vi "Facade.vi"(0 "Data In":T7 {"Duration (s)" format="%<%M:%S>T"}, 2 "Display State In":T5, 3 "Container State":T6) -> (6 "Data Out":T7 {"Duration (s)" format="%<%M:%S>T"}, 7 "Display State Out":T5, 8 "Action":T4)   [LabVIEW 2015, in "Artist Browser.lvlib" / "Artist Browser.xctl"]
uses:
  Artist Browser.xctl
  Data.ctl
  controls/Music Library Element Display.ctl
  file/MusicElement/Song/Song Duration.ctl
  <vilib>/_xctls/Container State.ctl
  State.ctl
  <vilib>/_xctls/Action.ctl
  controls/Ascending_Descending Order.ctl
  file/MusicElement/MusicElementLibrary/MusicLibrary/Music Library Sort Option.ctl
  <vilib>/_xctls/XControlSupport.lvlib
  file/MusicElement/MusicElementLibrary/MusicLibrary/MusicLibrary.lvclass
  file/MusicElement/Song/Song.lvclass
panel:
  out "Unfiltered Array":T1[](array[typedef]) {"Duration (s)" format="%<%M:%S>T"}
  in  "Remove Filters":bool
  in  "Time Sort":bool
  out "Sort Time Indicator":T3
  out "Sort Artist Indicator":T3
  in  "Artist Sort":bool
  in  "Song Sort":bool
  out "Sort Songs Indicator":T3
  in  "Array":T1[](array[typedef]) {"Duration (s)" format="%<%M:%S>T"}
  in  "Scrollbar":i32(c297)
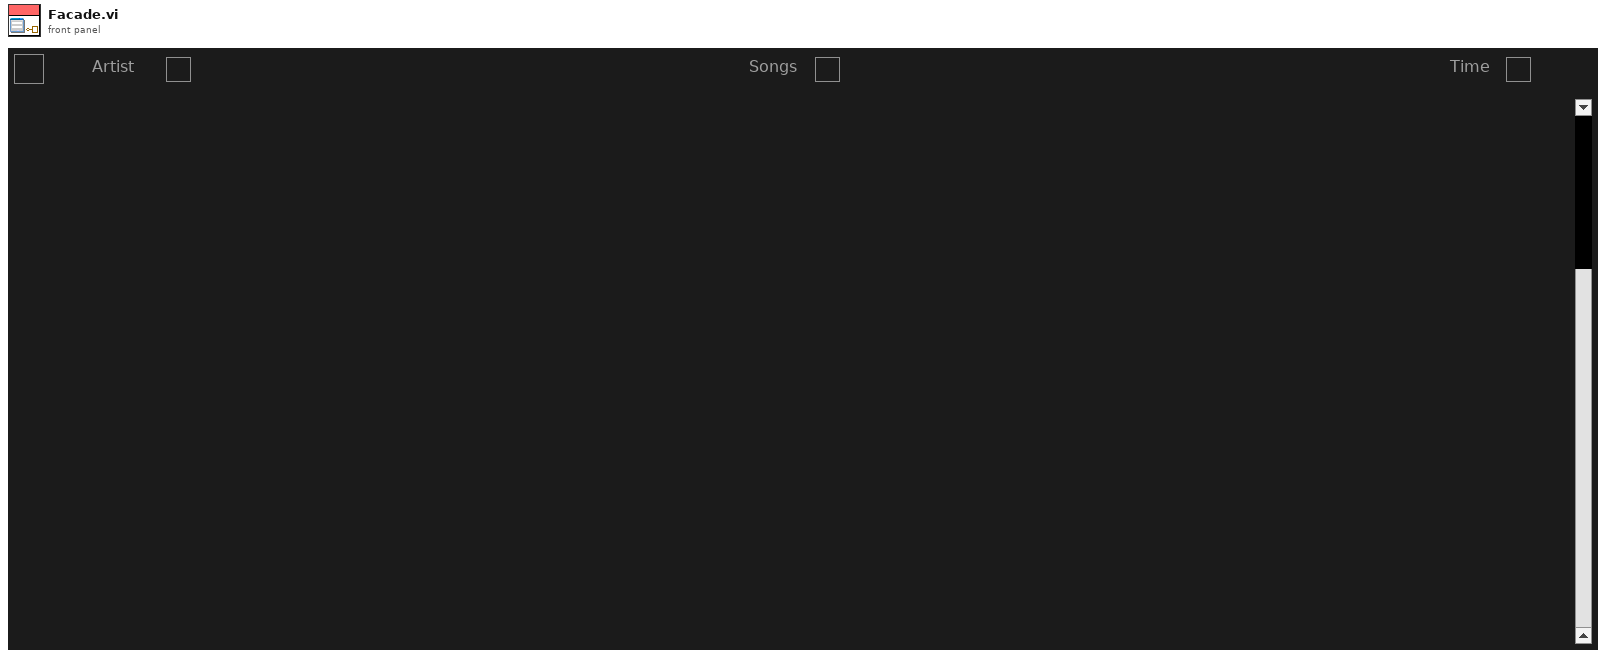
[diagram p1: front panel]
types:
  T1 = typedef "Music Library Element Display.ctl" = cluster{"Name":string, "Details":string, "Duration (s)":T2, "Click":bool}
  T2 = typedef "Song.lvclass/Song Duration.ctl" = timestamp
  T3 = typedef "Ascending_Descending Order.ctl" = bool
  T4 = typedef "XControlSupport.lvlib/Action.ctl" = cluster{"Data Changed?":bool, "State Changed?":bool, "Action Name":string}
  T5 = typedef "Artist Browser.lvlib/Artist Browser.xctl/State.ctl" = cluster{"Event - Element Selected":refnum<user-event>}
  T6 = typedef "XControlSupport.lvlib/Container State.ctl" = cluster{"Indicator?":bool, "Run Mode?":bool, " Refnum":refnum<vi>}
  T7 = typedef "Artist Browser.lvlib/Artist Browser.xctl/Data.ctl" = T1[]
  T8 = cluster{"Name":bool, "Details":bool, "Duration (s)":bool, "Click":bool}
  T9 = typedef "MusicLibrary.lvclass/Music Library Sort Option.ctl" = enum16{"Name", "Details", "Time"}
  T10 = cluster{"Name":bool, "Details":bool, "Duration (s)":bool, "Click":bool}[]
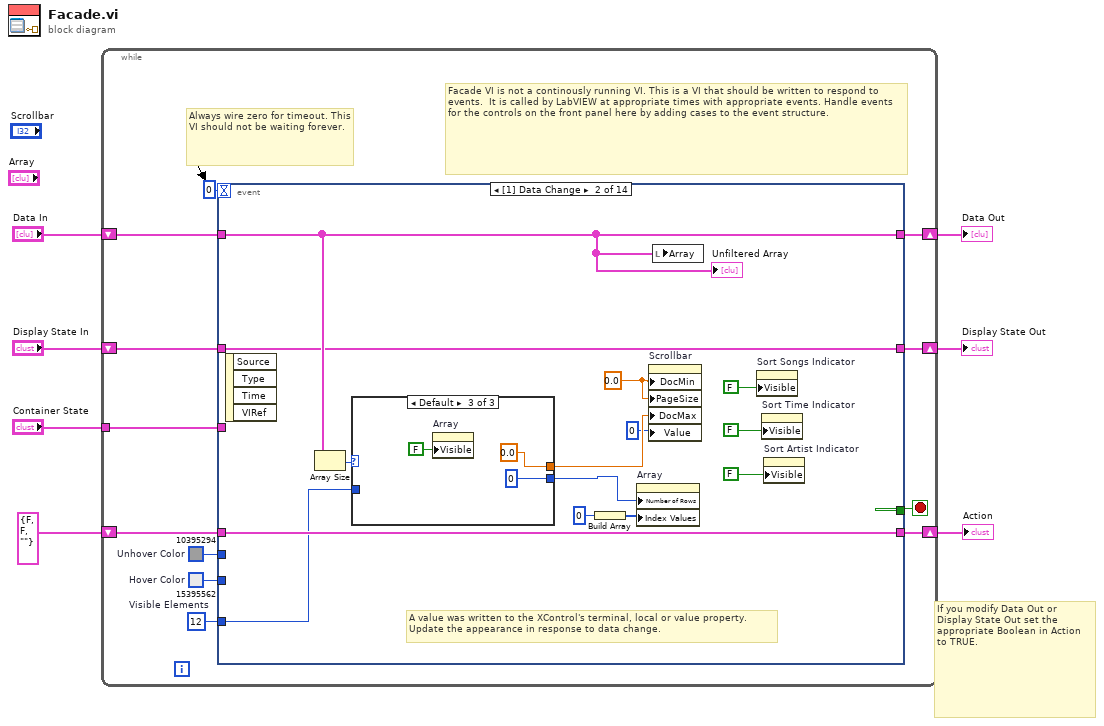
[diagram p0: block diagram]
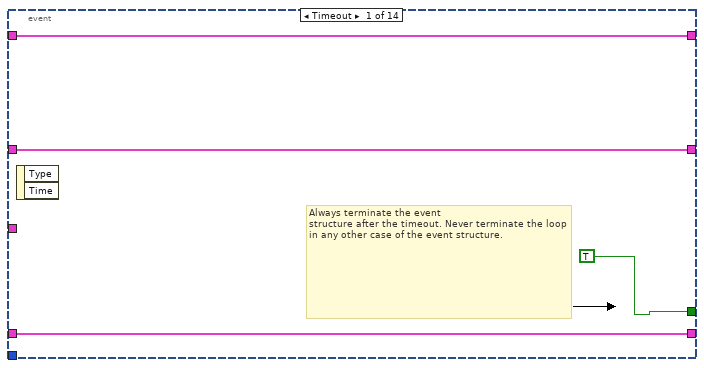
[diagram p2: hidden frame]
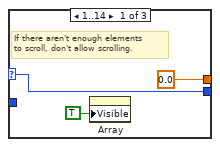
[diagram p3: hidden frame]
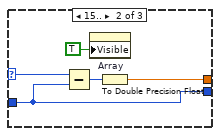
[diagram p4: hidden frame]
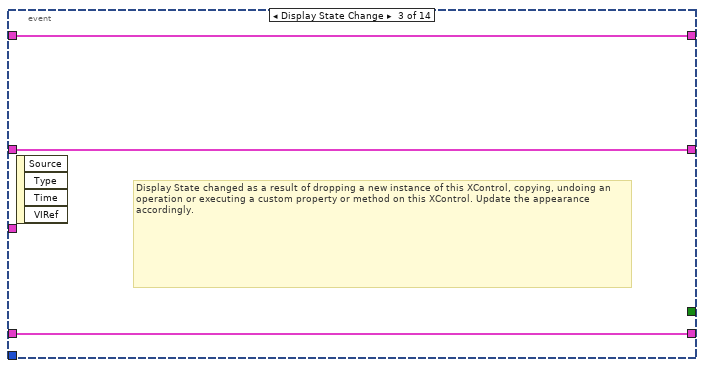
[diagram p5: hidden frame]
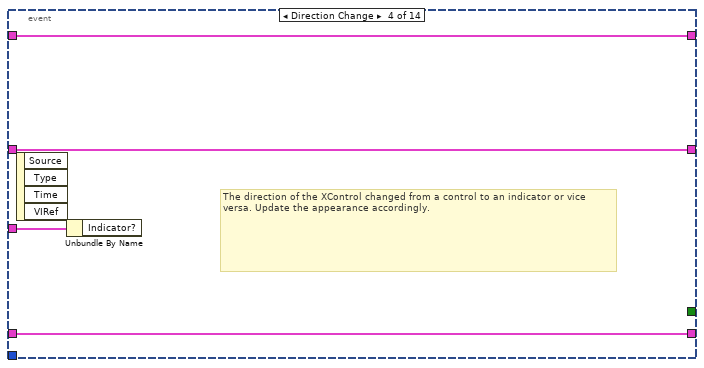
[diagram p6: hidden frame]
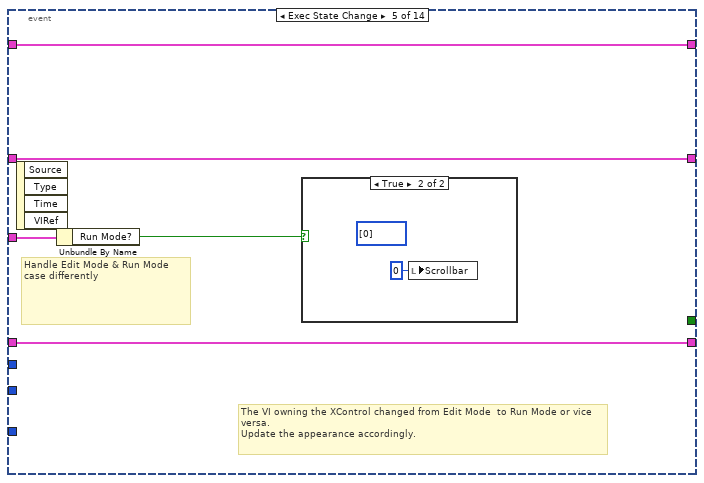
[diagram p7: hidden frame]
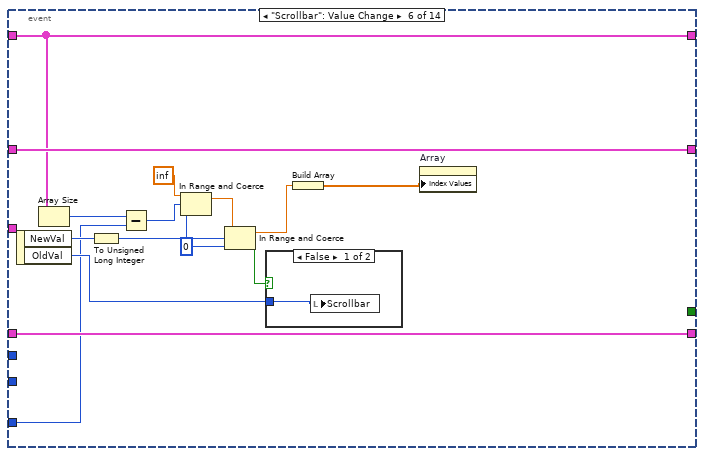
[diagram p9: hidden frame]
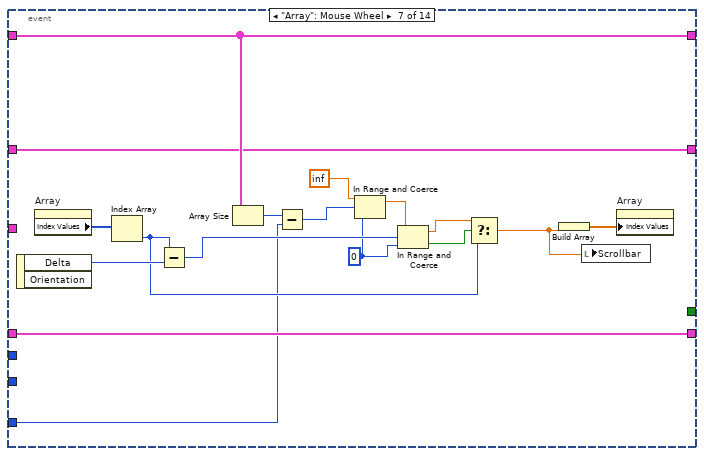
[diagram p11: hidden frame]
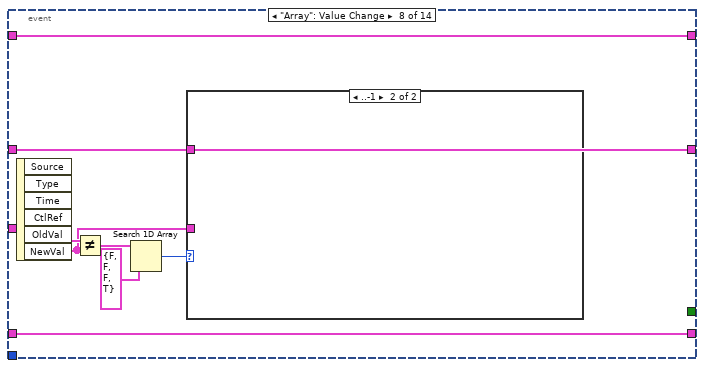
[diagram p12: hidden frame]
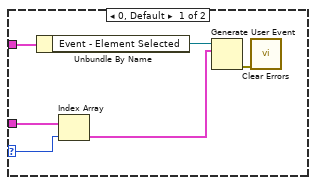
[diagram p13: hidden frame]
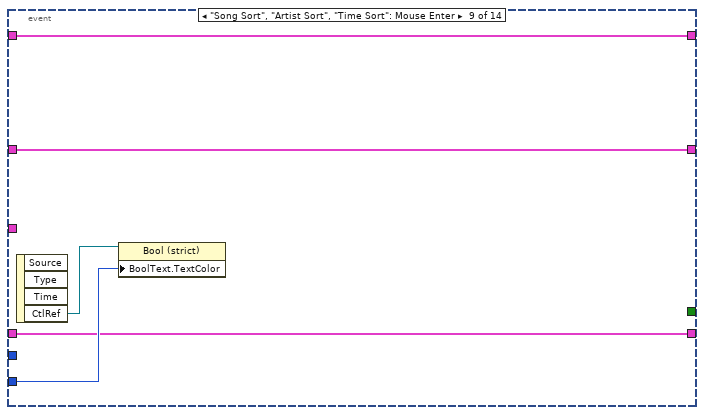
[diagram p14: hidden frame]
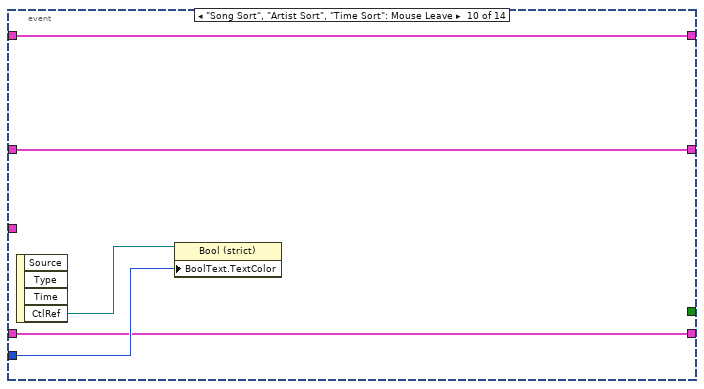
[diagram p15: hidden frame]
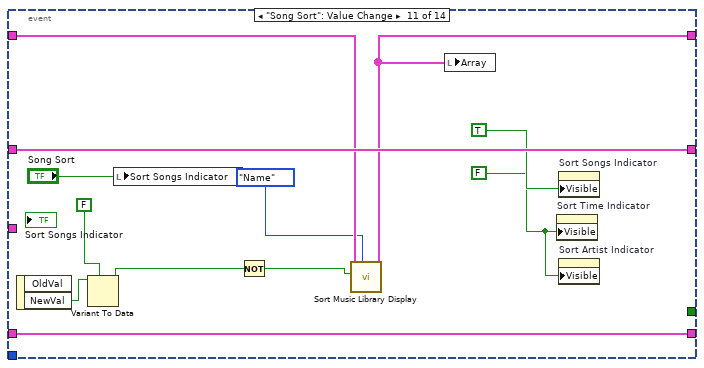
[diagram p16: hidden frame]
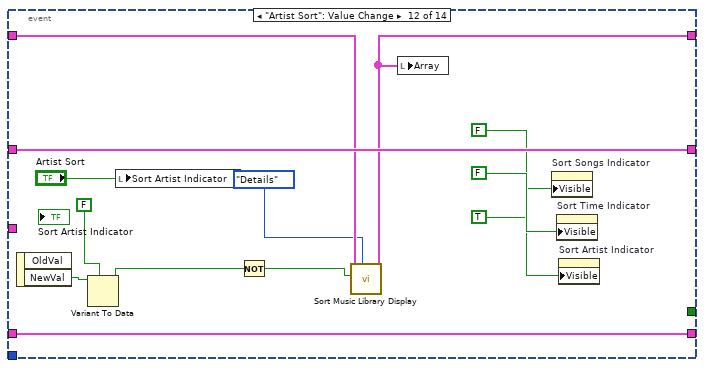
[diagram p17: hidden frame]
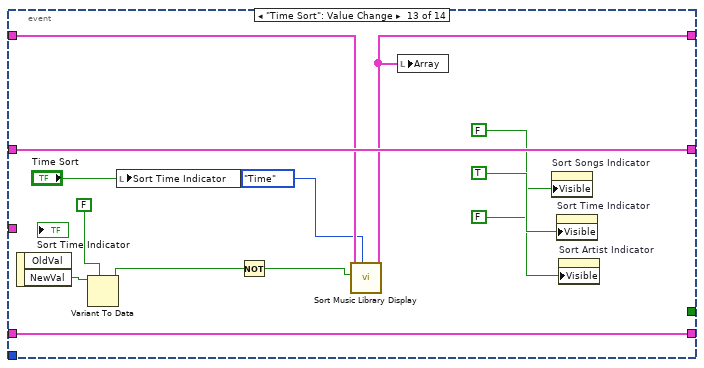
[diagram p18: hidden frame]
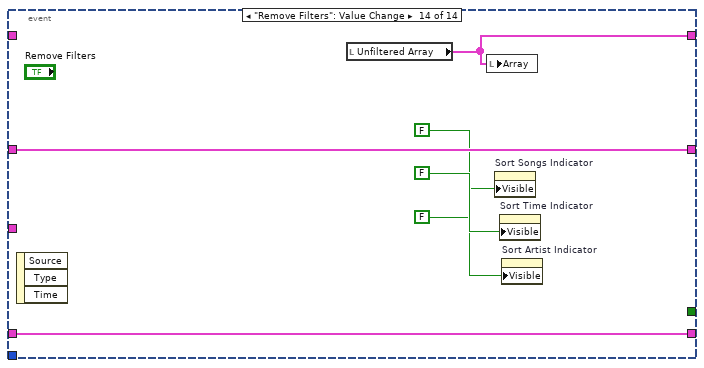
[diagram p19: hidden frame]
diagram:
  # "If you modify Data Out or\nDisplay State Out set the\nappropriate Boolean in Action\nto TRUE."
  n1 = while {
    shift-right: [w18] -> w3
    shift-left: "Display State In" -> [w19]
    tunnel: "Container State" -> [w15]
    shift-right: [w13] -> w2
    shift-left: "Data In" -> [w14]
    shift-right: [w11] -> w1
    shift-left: T4 {"Data Changed?"=FALSE, "State Changed?"=FALSE, "Action Name"=""} ("Action") -> [w12]
    stop <- w17 stop-if-true
    w8 = u32 15395562  # Hover Color
    w9 = u32 10395294  # Unhover Color
    w10 = 12  # Visible Elements
    # "Facade VI is not a continously running VI. This is a VI that should be written to respond to events.  It is called by LabVIEW at appropriate times with appropriate events. Handle events for the controls on the front panel here by adding cases to the event structure."
    # "Always wire zero for timeout. This\nVI should not be waiting forever."
    n2 = event shown="[1] Data Change" {
      selector: _ -> [_ _ _ _ _ _ _ _ _ _ _ _ _ _]
      dyn-events: _ -> [_ _ _ _ _ _ _ _ _ _ _ _ _ _]
      timeout: 0 -> [_ _ _ _ _ _ _ _ _ _ _ _ _ _]
      tunnel: w19 -> [w21 w27 w51 w54 w59 w74 w89 w95 w110 w115 w128 w142 w155 w162]
      tunnel: [w21 w27 w51 w54 w59 w74 w89 w95 w110 w115 w128 w142 w155 w162] -> w18
      tunnel: [TRUE _ _ _ _ _ _ _ _ _ _ _ _ _] -> w17
      tunnel: w15 -> [_ _ _ w55 w60 _ _ _ _ _ _ _ _ _]
      tunnel: w14 -> [w20 w28 w50 w53 w58 w72 w90 w102 w111 w114 w122 w134 w147 _]
      tunnel: [w20 w28 w50 w53 w58 w72 w90 w102 w111 w114 w121 w133 w146 w157] -> w13
      tunnel: [w22 w37 w49 w52 w57 w75 w91 w101 w109 w116 w127 w141 w154 w161] -> w11
      tunnel: w12 -> [w22 w37 w49 w52 w57 w75 w91 w101 w109 w116 w127 w141 w154 w161]
      tunnel: w10 -> [_ w35 _ _ _ w67 w85 _ _ _ _ _ _ _]
      tunnel: w9 -> [_ _ _ _ _ _ _ _ _ w117 _ _ _ _]
      tunnel: w8 -> [_ _ _ _ _ _ _ _ w112 _ _ _ _ _]
      event Timeout {
        # "Always terminate the event\nstructure after the timeout. Never terminate the loop in any other case of the event structure."
        n3 = event-data() -> ()  [unwired: 1 in, 2 out]
      }
      event Data Change {
        w31 = 0.0 ("Doc Min")
        # "A value was written to the XControl's terminal, local or value property.\nUpdate the appearance in response to data change."
        n4 = event-data() -> ()  [unwired: 1 in, 4 out]
        n5 = Array Size(array=w28) -> (size(s)=w36:i32)
        n6 = case shown="Default" w36 {
          selector: w36 -> [w40 w44 _]
          tunnel: [w40 w42 0 ("y")] -> w29
          tunnel: [0.0 ("Doc Min") w45 0.0 ("Doc Max")] -> w30
          tunnel: w35 -> [_ w42 _]
          frame 1..14 {
            # "If there aren't enough elements\nto scroll, don't allow scrolling."
            n7 = property on="Array" class="Arr (strict)"("Visible"=TRUE) -> ()  [unwired: 2 in, 2 out]
          }
          frame 15.. {
            n8 = Subtract(x=w44, y=w42) -> (x-y=w43:i32)
            n9 = property on="Array" class="Arr (strict)"("Visible"=TRUE) -> ()  [unwired: 2 in, 2 out]
            n10 = To Double Precision Float(number=w43) -> (double precision float=w45:dbl)
          }
          frame Default {
            n11 = property on="Array" class="Arr (strict)"("Visible"=FALSE) -> ()  [unwired: 2 in, 2 out]
          }
        }
        n12 = Build Array(0 ("y")) -> (w25:i32[])
        n13 = property on="Array" class="Arr (strict)"("Number of Rows"=w29, "Index Values"=w25) -> ()  [unwired: 2 in, 2 out]
        n14 = property on="Scrollbar" class="Scroll (strict)"("DocMin"=w31, "PageSize"=w31, "DocMax"=w30, "Value"=0 ("y")) -> ()  [unwired: 2 in, 2 out]
        n15 = local write "Array"(w28) -> ()
        n16 = property on="Sort Songs Indicator" class="Bool (strict)"("Visible"=FALSE) -> ()  [unwired: 2 in, 2 out]
        n17 = property on="Sort Time Indicator" class="Bool (strict)"("Visible"=FALSE) -> ()  [unwired: 2 in, 2 out]
        n18 = property on="Sort Artist Indicator" class="Bool (strict)"("Visible"=FALSE) -> ()  [unwired: 2 in, 2 out]
        "Unfiltered Array" <- w28
      }
      event Display State Change {
        # "Display State changed as a result of dropping a new instance of this XControl, copying, undoing an operation or executing a custom property or method on this XControl. Update the appearance accordingly."
        n19 = event-data() -> ()  [unwired: 1 in, 4 out]
      }
      event Direction Change {
        # "The direction of the XControl changed from a control to an indicator or vice versa. Update the appearance accordingly."
        n20 = event-data() -> ()  [unwired: 1 in, 4 out]
        n21 = Unbundle By Name(w55) -> ()  [unwired: 1 out]
      }
      event Exec State Change {
        # "The VI owning the XControl changed from Edit Mode  to Run Mode or vice versa.\nUpdate the appearance accordingly."
        # "Handle Edit Mode & Run Mode\ncase differently"
        n22 = event-data() -> ()  [unwired: 1 in, 4 out]
        n23 = Unbundle By Name(w60) -> ("Run Mode?"=w56:bool)
        n24 = case shown="True" w56 {
          frame False {
          }
          frame True {
            (unwired) u32[] [0] ("Index Values")
            n25 = local write "Scrollbar"(0 ("Scrollbar")) -> ()
          }
        }
      }
      event "Scrollbar": Value Change {
        w62 = u32 0 ("upper limit")
        n26 = event-data() -> ("NewVal"=w76:i32, "OldVal"=w68:i32)  [unwired: 1 in]
        n27 = Array Size(array=w72) -> (size(s)=w71:i32)
        n28 = To Unsigned Long Integer(number=w76) -> (unsigned 32bit integer=w73:u32)
        n29 = Subtract(x=w71, y=w67) -> (x-y=w64:i32)
        n30 = In Range and Coerce(upper limit=inf, x=w64, lower limit=w62) -> (coerced(x)=w63:dbl)  [unwired: 1 out]
        n31 = In Range and Coerce(upper limit=w63, x=w73, lower limit=w62) -> (coerced(x)=w70:dbl, In Range?=w69:bool)
        n32 = case shown="False" w69 {
          tunnel: w68 -> [w77 _]
          frame False {
            n33 = local write "Scrollbar"(w77) -> ()
          }
          frame True {
          }
        }
        n34 = Build Array(w70) -> (w66:dbl[])
        n35 = property on="Array" class="Arr (strict)"("Index Values"=w66) -> ()  [unwired: 2 in, 2 out]
      }
      event "Array": Mouse Wheel {
        w80 = u32 0 ("upper limit")
        n36 = event-data() -> ("Delta"=w94:i32)  [unwired: 1 in, 1 out]
        n37 = property on="Array" class="Arr (strict)"() -> ("Index Values"=w82:u32[])  [unwired: 2 in, 2 out]
        n38 = Index Array(array=w82) -> (element=w86:u32)  [unwired: 1 in]
        n39 = Subtract(x=w86, y=w94) -> (x-y=w92:u32)
        n40 = Array Size(array=w90) -> (size(s)=w93:i32)
        n41 = Subtract(x=w93, y=w85) -> (x-y=w79:i32)
        n42 = In Range and Coerce(upper limit=inf, x=w79, lower limit=w80) -> (coerced(x)=w78:dbl)  [unwired: 1 out]
        n43 = In Range and Coerce(upper limit=w78, x=w92, lower limit=w80) -> (coerced(x)=w87:dbl, In Range?=w88:bool)
        n44 = Select(t=w87, s=w88, f=w86) -> (s? t:f=w84:dbl)
        n45 = Build Array(w84) -> (w83:dbl[])
        n46 = local write "Scrollbar"(w84) -> ()
        n47 = property on="Array" class="Arr (strict)"("Index Values"=w83) -> ()  [unwired: 2 in, 2 out]
      }
      event "Array": Value Change {
        n48 = event-data() -> ("OldVal"=w99:T1[], "NewVal"=w96:T1[])  [unwired: 1 in, 4 out]
        n49 = Not Equal?(x=w99, y=w96) -> (x != y?=w98:T10)
        n50 = Search 1D Array(1D array=w98, element=T8 {"Name"=FALSE, "Details"=FALSE, "Duration (s)"=FALSE, "Click"=TRUE}) -> (index of element=w97:i32)  [unwired: 1 in]
        n51 = case shown="..-1" w97 {
          selector: w97 -> [w106 _]
          tunnel: w95 -> [w108 _]
          tunnel: w96 -> [w105 _]
          frame 0, Default {
            n52 = Unbundle By Name(w108) -> ("Event - Element Selected"=w104:refnum<user-event>)
            n53 = Index Array(array=w105, index=w106) -> (element=w103:T1)
            n54 = Generate User Event(user event=w104, event data cluster=w103) -> (error out=w107:errorcluster)  [unwired: 2 in, 1 out]
            n55 = call <vilib>:"Clear Errors.vi"("error in (no error)"=w107) -> ()  [unwired: 5 in, 2 out]
          }
          frame ..-1 {
          }
        }
      }
      event "Song Sort", "Artist Sort", "Time Sort": Mouse Enter {
        n56 = event-data() -> ("CtlRef"=w113:refnum<vi>)  [unwired: 1 in, 3 out]
        n57 = property class="Bool (strict)"(reference=w113, "BoolText.TextColor"=w112) -> ()  [unwired: 1 in, 2 out]
      }
      event "Song Sort", "Artist Sort", "Time Sort": Mouse Leave {
        n58 = event-data() -> ("CtlRef"=w118:refnum<vi>)  [unwired: 1 in, 3 out]
        n59 = property class="Bool (strict)"(reference=w118, "BoolText.TextColor"=w117) -> ()  [unwired: 1 in, 2 out]
      }
      event "Song Sort": Value Change {
        w125 = FALSE ("Visible")
        n60 = event-data() -> ("NewVal"=w123:bool)  [unwired: 1 in, 1 out]
        n61 = Variant To Data(type=T3 FALSE ("Sort Songs Indicator"), Variant=w123) -> (data=w124:T3)  [unwired: 1 in, 1 out]
        n62 = local write "Sort Songs Indicator"("Song Sort") -> ()
        n63 = Not(x=w124) -> (.not. x?=w120:T3)
        n64 = call "Sort Music Library Display.vi"("Options"=Music_Library_Sort_Option."Name", "Reverse?"=w120, "Songs"=w122) -> ("Sorted Songs"=w121:T1[])  [unwired: 7 in, 1 out]
        n65 = local write "Array"(w121) -> ()
        n66 = property on="Sort Time Indicator" class="Bool (strict)"("Visible"=w125) -> ()  [unwired: 2 in, 2 out]
        n67 = property on="Sort Songs Indicator" class="Bool (strict)"("Visible"=TRUE) -> ()  [unwired: 2 in, 2 out]
        n68 = property on="Sort Artist Indicator" class="Bool (strict)"("Visible"=w125) -> ()  [unwired: 2 in, 2 out]
      }
      event "Artist Sort": Value Change {
        n69 = event-data() -> ("NewVal"=w135:bool)  [unwired: 1 in, 1 out]
        n70 = Variant To Data(type=T3 FALSE ("Sort Songs Indicator"), Variant=w135) -> (data=w139:T3)  [unwired: 1 in, 1 out]
        n71 = local write "Sort Artist Indicator"("Artist Sort") -> ()
        n72 = Not(x=w139) -> (.not. x?=w131:T3)
        n73 = call "Sort Music Library Display.vi"("Options"=Music_Library_Sort_Option."Details", "Reverse?"=w131, "Songs"=w134) -> ("Sorted Songs"=w133:T1[])  [unwired: 7 in, 1 out]
        n74 = local write "Array"(w133) -> ()
        n75 = property on="Sort Songs Indicator" class="Bool (strict)"("Visible"=FALSE) -> ()  [unwired: 2 in, 2 out]
        n76 = property on="Sort Time Indicator" class="Bool (strict)"("Visible"=FALSE) -> ()  [unwired: 2 in, 2 out]
        n77 = property on="Sort Artist Indicator" class="Bool (strict)"("Visible"=TRUE) -> ()  [unwired: 2 in, 2 out]
      }
      event "Time Sort": Value Change {
        n78 = event-data() -> ("NewVal"=w150:bool)  [unwired: 1 in, 1 out]
        n79 = Variant To Data(type=T3 FALSE ("Sort Songs Indicator"), Variant=w150) -> (data=w152:T3)  [unwired: 1 in, 1 out]
        n80 = local write "Sort Time Indicator"("Time Sort") -> ()
        n81 = Not(x=w152) -> (.not. x?=w145:T3)
        n82 = call "Sort Music Library Display.vi"("Options"=Music_Library_Sort_Option."Time", "Reverse?"=w145, "Songs"=w147) -> ("Sorted Songs"=w146:T1[])  [unwired: 7 in, 1 out]
        n83 = local write "Array"(w146) -> ()
        n84 = property on="Sort Songs Indicator" class="Bool (strict)"("Visible"=FALSE) -> ()  [unwired: 2 in, 2 out]
        n85 = property on="Sort Time Indicator" class="Bool (strict)"("Visible"=TRUE) -> ()  [unwired: 2 in, 2 out]
        n86 = property on="Sort Artist Indicator" class="Bool (strict)"("Visible"=FALSE) -> ()  [unwired: 2 in, 2 out]
      }
      event "Remove Filters": Value Change {
        n87 = event-data() -> ()  [unwired: 1 in, 3 out]
        n88 = local read "Unfiltered Array"() -> (w157:T1[])
        n89 = local write "Array"(w157) -> ()
        n90 = property on="Sort Songs Indicator" class="Bool (strict)"("Visible"=FALSE) -> ()  [unwired: 2 in, 2 out]
        n91 = property on="Sort Time Indicator" class="Bool (strict)"("Visible"=FALSE) -> ()  [unwired: 2 in, 2 out]
        n92 = property on="Sort Artist Indicator" class="Bool (strict)"("Visible"=FALSE) -> ()  [unwired: 2 in, 2 out]
      }
    }
  }
  "Display State Out" <- w3
  "Data Out" <- w2
  "Action" <- w1
